vi "Wait for Printing To Complete.vi"(8 "error in (no error)":errorcluster, 11 "File Name":string) -> (0 "error out":errorcluster)   [LabVIEW 2017]
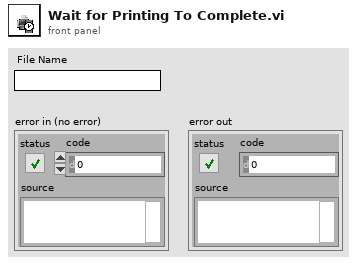
[diagram p1: front panel]
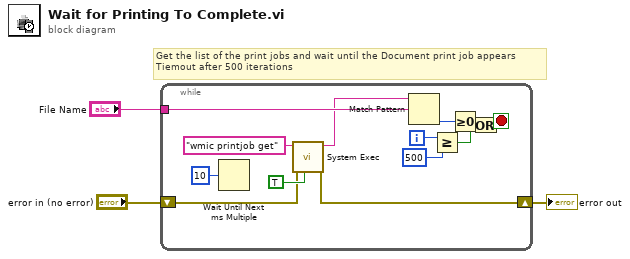
[diagram p0: block diagram]
diagram:
  # "Get the list of the print jobs and wait until the Document print job appears\nTiemout after 500 iterations"
  n1 = while {
    shift-right: [w12] -> w2
    shift-left: "error in (no error)" -> [w13]
    tunnel: "File Name" -> [w11]
    i -> [w8]
    stop <- w6 stop-if-true
    n2 = Wait Until Next ms Multiple(millisecond multiple=u32 10) -> ()  [unwired: 1 out]
    n3 = call <vilib>:"System Exec.vi"("run minimized? (F)"=TRUE, "error in (no error)"=w13, "command line"="wmic printjob get") -> ("error out"=w12:errorcluster, "standard output"=w4:string)  [unwired: 5 in, 2 out]
    n4 = Match Pattern(string=w4, regular expression=w11) -> (offset past match=w10:i32)  [unwired: 1 in, 3 out]
    n5 = Greater Or Equal?(x=w8, y=500) -> (x >= y?=w5:bool)
    n6 = Greater Or Equal To 0?(x=w10) -> (x >= 0?=w9:bool)
    n7 = Or(x=w9, y=w5) -> (x .or. y?=w6:bool)
  }
  "error out" <- w2
